vi "Add WebService.vi"() -> ()   [LabVIEW 2014]
panel:
  out "error out":errorcluster
  out "Array 3":path[](array[path])=[path "C:/Users/tom/Documents/programming/LabVIEW/FPPublisher/www/static", path "C:/Users/tom/Documents/programming/LabVIEW/FPPublisher/www/static/css", path "C:/Users/tom/Documents/programming/LabVIEW/FPPublisher/www/static/css/bootstrap-responsive.css", path "C:/Users/tom/Documents/programming/LabVIEW/FPPublisher/www/static/css/bootstrap-responsive.min.css", path "C:/Users/tom/Documents/programming/LabVIEW/FPPublisher/www/static/css/bootstrap.css", path "C:/Users/tom/Documents/programming/LabVIEW/FPPublisher/www/static/css/bootstrap.min.css", path "C:/Users/tom/Documents/programming/LabVIEW/FPPublisher/www/static/css/jquery.jqplot.min.css", path "C:/Users/tom/Documents/programming/LabVIEW/FPPublisher/www/static/img", path "C:/Users/tom/Documents/programming/LabVIEW/FPPublisher/www/static/img/glyphicons-halflings-white.png", path "C:/Users/tom/Documents/programming/LabVIEW/FPPublisher/www/static/img/glyphicons-halflings.png", path "C:/Users/tom/Documents/programming/LabVIEW/FPPublisher/www/static/img/Thumbs.db", path "C:/Users/tom/Documents/programming/LabVIEW/FPPublisher/www/static/img/UID467_1.png", path "C:/Users/tom/Documents/programming/LabVIEW/FPPublisher/www/static/img/UID467_2.png", path "C:/Users/tom/Documents/programming/LabVIEW/FPPublisher/www/static/img/UID678_1.png", path "C:/Users/tom/Documents/programming/LabVIEW/FPPublisher/www/static/img/UID678_2.png", path "C:/Users/tom/Documents/programming/LabVIEW/FPPublisher/www/static/js", path "C:/Users/tom/Documents/programming/LabVIEW/FPPublisher/www/static/js/jquery-ui", path "C:/Users/tom/Documents/programming/LabVIEW/FPPublisher/www/static/js/jquery-ui/external", path "C:/Users/tom/Documents/programming/LabVIEW/FPPublisher/www/static/js/jquery-ui/external/jquery", path "C:/Users/tom/Documents/programming/LabVIEW/FPPublisher/www/static/js/jquery-ui/external/jquery/jquery.js", path "C:/Users/tom/Documents/programming/LabVIEW/FPPublisher/www/static/js/jquery-ui/images", path "C:/Users/tom/Documents/programming/LabVIEW/FPPublisher/www/static/js/jquery-ui/images/ui-bg_flat_0_aaaaaa_40x100.png", path "C:/Users/tom/Documents/programming/LabVIEW/FPPublisher/www/static/js/jquery-ui/images/ui-bg_flat_75_ffffff_40x100.png", path "C:/Users/tom/Documents/programming/LabVIEW/FPPublisher/www/static/js/jquery-ui/images/ui-bg_glass_55_fbf9ee_1x400.png", path "C:/Users/tom/Documents/programming/LabVIEW/FPPublisher/www/static/js/jquery-ui/images/ui-bg_glass_65_ffffff_1x400.png", path "C:/Users/tom/Documents/programming/LabVIEW/FPPublisher/www/static/js/jquery-ui/images/ui-bg_glass_75_dadada_1x400.png", path "C:/Users/tom/Documents/programming/LabVIEW/FPPublisher/www/static/js/jquery-ui/images/ui-bg_glass_75_e6e6e6_1x400.png", path "C:/Users/tom/Documents/programming/LabVIEW/FPPublisher/www/static/js/jquery-ui/images/ui-bg_glass_95_fef1ec_1x400.png", path "C:/Users/tom/Documents/programming/LabVIEW/FPPublisher/www/static/js/jquery-ui/images/ui-bg_highlight-soft_75_cccccc_1x100.png", path "C:/Users/tom/Documents/programming/LabVIEW/FPPublisher/www/static/js/jquery-ui/images/ui-icons_2e83ff_256x240.png", path "C:/Users/tom/Documents/programming/LabVIEW/FPPublisher/www/static/js/jquery-ui/images/ui-icons_222222_256x240.png", path "C:/Users/tom/Documents/programming/LabVIEW/FPPublisher/www/static/js/jquery-ui/images/ui-icons_454545_256x240.png", path "C:/Users/tom/Documents/programming/LabVIEW/FPPublisher/www/static/js/jquery-ui/images/ui-icons_888888_256x240.png", path "C:/Users/tom/Documents/programming/LabVIEW/FPPublisher/www/static/js/jquery-ui/images/ui-icons_cd0a0a_256x240.png", path "C:/Users/tom/Documents/programming/LabVIEW/FPPublisher/www/static/js/jquery-ui/index.html", path "C:/Users/tom/Documents/programming/LabVIEW/FPPublisher/www/static/js/jquery-ui/jquery-ui.css", path "C:/Users/tom/Documents/programming/LabVIEW/FPPublisher/www/static/js/jquery-ui/jquery-ui.js", path "C:/Users/tom/Documents/programming/LabVIEW/FPPublisher/www/static/js/jquery-ui/jquery-ui.min.css", path "C:/Users/tom/Documents/programming/LabVIEW/FPPublisher/www/static/js/jquery-ui/jquery-ui.min.js", path "C:/Users/tom/Documents/programming/LabVIEW/FPPublisher/www/static/js/jquery-ui/jquery-ui.structure.css", path "C:/Users/tom/Documents/programming/LabVIEW/FPPublisher/www/static/js/jquery-ui/jquery-ui.structure.min.css", path "C:/Users/tom/Documents/programming/LabVIEW/FPPublisher/www/static/js/jquery-ui/jquery-ui.theme.css", path "C:/Users/tom/Documents/programming/LabVIEW/FPPublisher/www/static/js/jquery-ui/jquery-ui.theme.min.css", path "C:/Users/tom/Documents/programming/LabVIEW/FPPublisher/www/static/js/bootstrap.js", path "C:/Users/tom/Documents/programming/LabVIEW/FPPublisher/www/static/js/bootstrap.min.js", path "C:/Users/tom/Documents/programming/LabVIEW/FPPublisher/www/static/js/jqplot.canvasAxisLabelRenderer.min.js", path "C:/Users/tom/Documents/programming/LabVIEW/FPPublisher/www/static/js/jqplot.canvasTextRenderer.min.js", path "C:/Users/tom/Documents/programming/LabVIEW/FPPublisher/www/static/js/jqplot.categoryAxisRenderer.min.js", path "C:/Users/tom/Documents/programming/LabVIEW/FPPublisher/www/static/js/jquery.jqplot.js", path "C:/Users/tom/Documents/programming/LabVIEW/FPPublisher/www/static/js/jquery.jqplot.min.js", path "C:/Users/tom/Documents/programming/LabVIEW/FPPublisher/www/static/js/jquery.min.js", path "C:/Users/tom/Documents/programming/LabVIEW/FPPublisher/www/static/js/Main.js", path "C:/Users/tom/Documents/programming/LabVIEW/FPPublisher/www/static/js/Simple.js", path "C:/Users/tom/Documents/programming/LabVIEW/FPPublisher/www/static/favicon.ico", path "C:/Users/tom/Documents/programming/LabVIEW/FPPublisher/www/static/Main.html", path "C:/Users/tom/Documents/programming/LabVIEW/FPPublisher/www/static/Simple.html", path "", path "C:/Users/tom/Documents/programming/LabVIEW/FPPublisher/FPServer.vi", path "", path "C:/Users/tom/Documents/programming/LabVIEW/FPPublisher/www/GetData.vi", path "C:/Users/tom/Documents/programming/LabVIEW/FPPublisher/www/SetData.vi"]
  out "Array 2":string[](array[string])=["Folder", "Folder", "Document", "Document", "Document", "Document", "Document", "Folder", "Document", "Document", "Document", "Document", "Document", "Document", "Document", "Folder", "Folder", "Folder", "Folder", "Document", "Folder", "Document", "Document", "Document", "Document", "Document", "Document", "Document", "Document", "Document", "Document", "Document", "Document", "Document", "Document", "Document", "Document", "Document", "Document", "Document", "Document", "Document", "Document", "Document", "Document", "Document", "Document", "Document", "Document", "Document", "Document", "Document", "Document", "Document", "Document", "Document", "Startup VIs Container", "VI", "HTTP WebResources Container", "VI", "VI"]
  out "Array":string[](array[string])=["Public Content", "css", "bootstrap-responsive.css", "bootstrap-responsive.min.css", "bootstrap.css", "bootstrap.min.css", "jquery.jqplot.min.css", "img", "glyphicons-halflings-white.png", "glyphicons-halflings.png", "Thumbs.db", "UID467_1.png", "UID467_2.png", "UID678_1.png", "UID678_2.png", "js", "jquery-ui", "external", "jquery", "jquery.js", "images", "ui-bg_flat_0_aaaaaa_40x100.png", "ui-bg_flat_75_ffffff_40x100.png", "ui-bg_glass_55_fbf9ee_1x400.png", "ui-bg_glass_65_ffffff_1x400.png", "ui-bg_glass_75_dadada_1x400.png", "ui-bg_glass_75_e6e6e6_1x400.png", "ui-bg_glass_95_fef1ec_1x400.png", "ui-bg_highlight-soft_75_cccccc_1x100.png", "ui-icons_2e83ff_256x240.png", "ui-icons_222222_256x240.png", "ui-icons_454545_256x240.png", "ui-icons_888888_256x240.png", "ui-icons_cd0a0a_256x240.png", "index.html", "jquery-ui.css", "jquery-ui.js", "jquery-ui.min.css", "jquery-ui.min.js", "jquery-ui.structure.css", "jquery-ui.structure.min.css", "jquery-ui.theme.css", "jquery-ui.theme.min.css", "bootstrap.js", "bootstrap.min.js", "jqplot.canvasAxisLabelRenderer.min.js", "jqplot.canvasTextRenderer.min.js", "jqplot.categoryAxisRenderer.min.js", "jquery.jqplot.js", "jquery.jqplot.min.js", "jquery.min.js", "Main.js", "Simple.js", "favicon.ico", "Main.html", "Simple.html", "Startup VIs", "FPServer.vi", "Web Resources", "GetData.vi", "SetData.vi"]
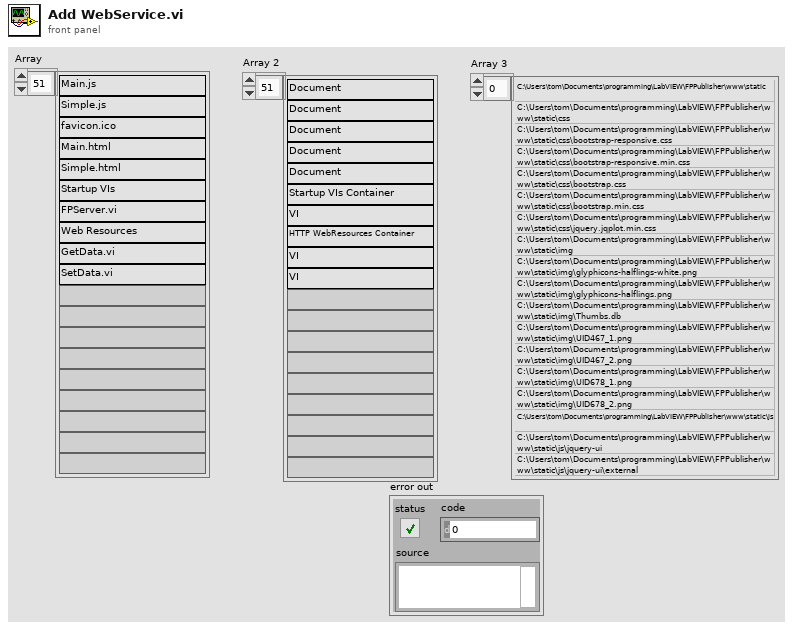
[diagram p1: front panel]
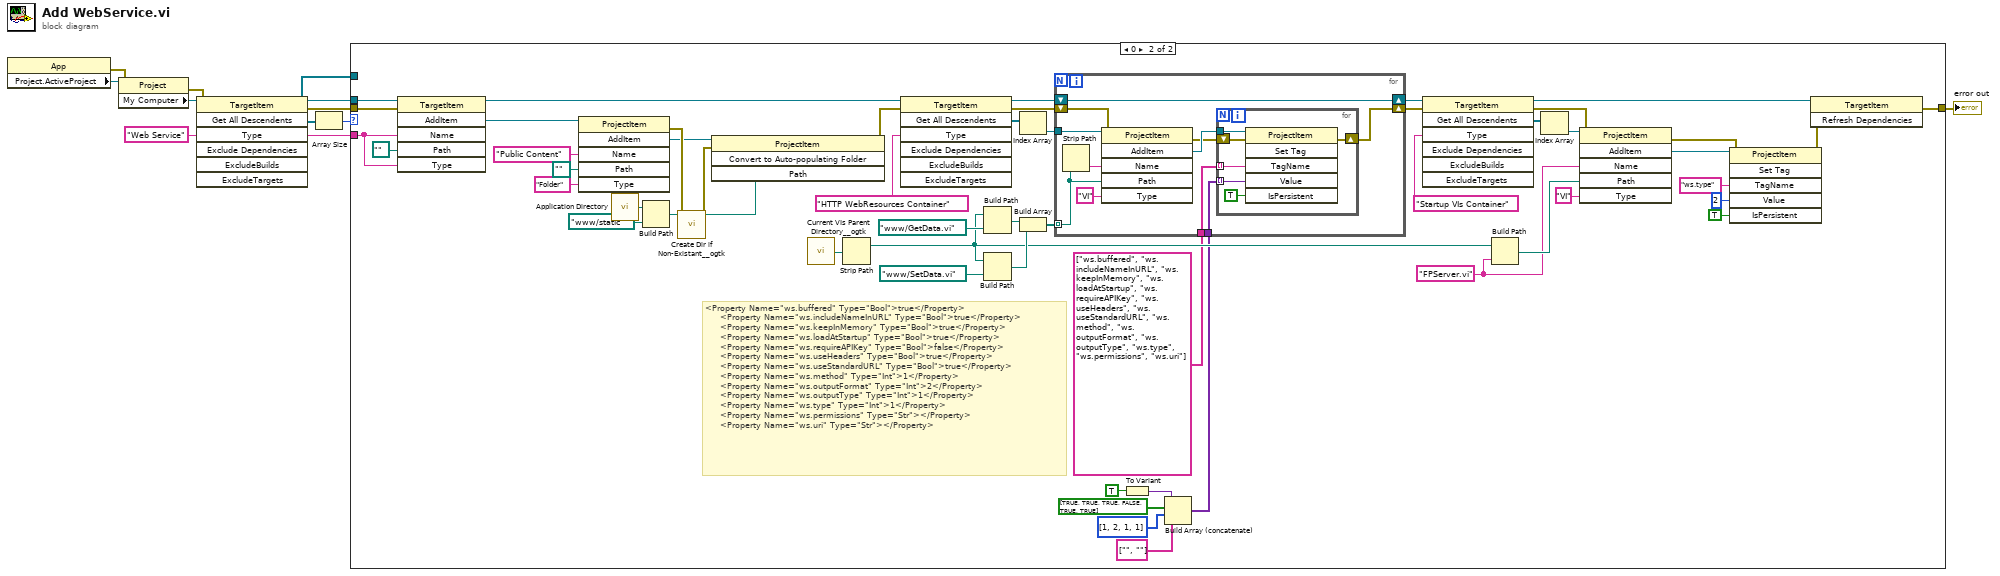
[diagram p0: block diagram]
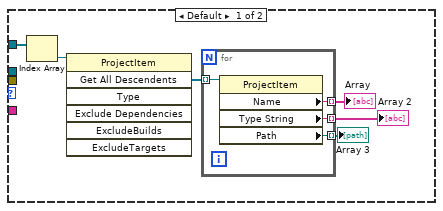
[diagram p2: hidden frame]
diagram:
  w4 = "Web Service" ("Type")
  n1 = property class="App"() -> (error out=w10:errorcluster, "Project.ActiveProject"=w7:refnum<vi>)  [unwired: 2 in, 1 out]
  n2 = property class="Project"(reference=w7, error in=w10) -> (error out=w9:errorcluster, "My Computer"=w6:refnum<vi>)  [unwired: 1 out]
  n3 = invoke class="TargetItem" method="Get All Descendents"(reference=w6, error in=w9, "Type"=w4) -> (reference out=w5:refnum<vi>, error out=w8:errorcluster, "All Descendents"=w2:refnum<vi>[])  [unwired: 4 in, 4 out]
  n4 = Array Size(array=w2) -> (size(s)=w3:i32)
  n5 = case shown="0" w3 {
    tunnel: w5 -> [_ w70]
    tunnel: w4 -> [_ w69]
    tunnel: w2 -> [w16 _]
    tunnel: w8 -> [_ w73]
    tunnel: [_ w34] -> w1
    frame Default {
      n6 = Index Array(array=w16) -> (element=w15:refnum<vi>)  [unwired: 1 in]
      n7 = invoke class="ProjectItem" method="Get All Descendents"(reference=w15) -> ("All Descendents"=w14:refnum<vi>[])  [unwired: 6 in, 6 out]
      n8 = for {
        tunnel: w14 -> [w20] mode=indexing
        tunnel: [w19] -> w13 mode=indexing
        tunnel: [w18] -> w12 mode=indexing
        tunnel: [w17] -> w11 mode=indexing
        n9 = property class="ProjectItem"(reference=w20) -> ("Name"=w19:string, "Type String"=w18:string, "Path"=w17:path)  [unwired: 1 in, 2 out]
      }
      "Array" <- w13
      "Array 2" <- w12
      "Array 3" <- w11
    }
    frame 0 {
      w39 = "FPServer.vi" ("Path")
      # "<Property Name=\"ws.buffered\" Type=\"Bool\">true</Property>\n\t\t\t\t\t<Property Name=\"ws.includeNameInURL\" Type=\"Bool\">true</Property>\n\t\t\t\t\t<Property Name=\"ws.keepInMemory\" Type=\"Bool\">true</Property>\n\t\t\t\t\t<Property Name=\"ws.loadAtStartup\" Type=\"Bool\">true</Property>\n\t\t\t\t\t<Property Name=\"ws.requireAPIKey\" Type=\"Bool\">false</Property>\n\t\t\t\t\t<Property Name=\"ws.useHeaders\" Type=\"Bool\">true</Property>\n\t\t\t\t\t<Property Name=\"ws.useStandardURL\" Type=\"Bool\">true</Property>\n\t\t\t\t\t<Property Name=\"ws.method\" Type=\"Int\">1</Property>\n\t\t\t\t\t<Property Name=\"ws.outputFormat\" Type=\"Int\">2</Property>\n\t\t\t\t\t<Property Name=\"ws.outputType\" Type=\"Int\">1</Property>\n\t\t\t\t\t<Property Name=\"ws.type\" Type=\"Int\">1</Property>\n\t\t\t\t\t<Property Name=\"ws.permissions\" Type=\"Str\"></Property>\n\t\t\t\t\t<Property Name=\"ws.uri\" Type=\"Str\"></Property>"
      n10 = invoke class="TargetItem" method="AddItem"(reference=w70, error in=w73, "Name"=w69, "Path"=path "", "Type"=w69) -> (reference out=w49:refnum<vi>, "AddItem"=w63:refnum<vi>)  [unwired: 1 in, 4 out]
      n11 = invoke class="ProjectItem" method="AddItem"(reference=w63, "Name"="Public Content" ("Type"), "Path"=path "", "Type"="Folder") -> (error out=w72:errorcluster, "AddItem"=w62:refnum<vi>)  [unwired: 2 in, 4 out]
      n12 = call <vilib>:"Application Directory.vi"() -> ("Application Directory"=w66:path)
      n13 = Build Path(base path=w66, name or relative path=path "www/static" ("Path")) -> (appended path=w64:path)
      n14 = call <userlib>:"Create Dir if Non-Existant__ogtk.vi"("error in (no error)"=w72, "Directory Path"=w64) -> ("error out"=w71:errorcluster, "dup Directory Path"=w56:path)  [unwired: 7 in, 1 out]
      n15 = invoke class="ProjectItem" method="Convert to Auto-populating Folder"(reference=w62, error in=w71, "Path"=w56) -> (error out=w48:errorcluster)  [unwired: 1 in, 3 out]
      n16 = call <userlib>:"Current VIs Parent Directory__ogtk.vi"() -> ("Parent Directory (+ Relative)"=w54:path)  [unwired: 5 in]
      n17 = Strip Path(path=w54) -> (stripped path=w42:path)  [unwired: 1 out]
      n18 = invoke class="TargetItem" method="Get All Descendents"(reference=w49, error in=w48, "Type"="HTTP WebResources Container") -> (reference out=w47:refnum<vi>, error out=w57:errorcluster, "All Descendents"=w58:refnum<vi>[])  [unwired: 4 in, 4 out]
      n19 = Build Path(base path=w42, name or relative path=path "www/GetData.vi" ("Path")) -> (appended path=w53:path)
      n20 = Build Path(base path=w42, name or relative path=path "www/SetData.vi" ("Path")) -> (appended path=w50:path)
      n21 = Index Array(array=w58) -> (element=w37:refnum<vi>)  [unwired: 1 in]
      n22 = Build Array(w53, w50) -> (w55:path[])
      n23 = To Variant(anything=TRUE) -> (Variant=w23:variant)
      n24 = Build Array (concatenate)(w23, bool[] [TRUE, TRUE, TRUE, FALSE, TRUE, TRUE], i32[] [1, 2, 1, 1], string[] ["", ""]) -> (w27:variant[])
      n25 = for {
        tunnel: w55 -> [w80] mode=indexing
        tunnel: w37 -> [w84]
        shift-right: [w76] -> w45
        shift-left: w57 -> [w79]
        shift-right: [w81] -> w46
        shift-left: w47 -> [w81]
        tunnel: string[] ["ws.buffered", "ws.includeNameInURL", "ws.keepInMemory", "ws.loadAtStartup", "ws.requireAPIKey", "ws.useHeaders", "ws.useStandardURL", "ws.method", "ws.outputFormat", "ws.outputType", "ws.type", "ws.permissions", "ws.uri"] -> [w75]
        tunnel: w27 -> [w74]
        n26 = Strip Path(path=w80) -> (name=w83:string)  [unwired: 1 out]
        n27 = invoke class="ProjectItem" method="AddItem"(reference=w84, error in=w79, "Name"=w83, "Path"=w80, "Type"="VI") -> (error out=w77:errorcluster, "AddItem"=w78:refnum<vi>)  [unwired: 1 in, 4 out]
        n28 = for {
          tunnel: w78 -> [w90]
          shift-right: [w88] -> w76
          shift-left: w77 -> [w89]
          tunnel: w75 -> [w87] mode=indexing
          tunnel: w74 -> [w86] mode=indexing
          n29 = invoke class="ProjectItem" method="Set Tag"(reference=w90, error in=w89, "TagName"=w87, "Value"=w86, "IsPersistent"=TRUE ("Is Persistent")) -> (error out=w88:errorcluster)  [unwired: 1 in, 5 out]
        }
      }
      n30 = invoke class="TargetItem" method="Get All Descendents"(reference=w46, error in=w45, "Type"="Startup VIs Container") -> (reference out=w35:refnum<vi>, error out=w38:errorcluster, "All Descendents"=w43:refnum<vi>[])  [unwired: 4 in, 4 out]
      n31 = Build Path(base path=w42, name or relative path=w39) -> (appended path=w41:path)
      n32 = Index Array(array=w43) -> (element=w36:refnum<vi>)  [unwired: 1 in]
      n33 = invoke class="ProjectItem" method="AddItem"(reference=w36, error in=w38, "Name"=w39, "Path"=w41, "Type"="VI") -> (error out=w29:errorcluster, "AddItem"=w33:refnum<vi>)  [unwired: 1 in, 4 out]
      n34 = invoke class="ProjectItem" method="Set Tag"(reference=w33, error in=w29, "TagName"="ws.type" ("Tag Name"), "Value"=2, "IsPersistent"=TRUE ("Is Persistent")) -> (error out=w28:errorcluster)  [unwired: 1 in, 5 out]
      n35 = invoke class="TargetItem" method="Refresh Dependencies"(reference=w35, error in=w28) -> (error out=w34:errorcluster)  [unwired: 1 in, 2 out]
    }
  }
  "error out" <- w1
